vi "AddCalanderToFrontPanel.vi"() -> ()   [LabVIEW 2019]
panel:
  out "To Date  2":string
  out "To Date":string
  in  "To Date Time":timestamp
  in  "From Date Time":timestamp
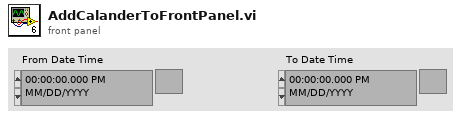
[diagram p1: front panel]
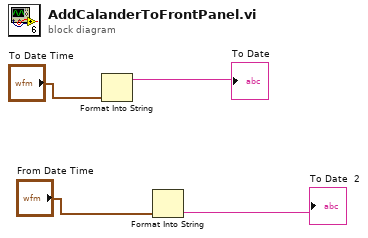
[diagram p0: block diagram]
diagram:
  n1 = Format Into String("To Date Time") -> (resulting string=→"To Date":string)  [unwired: 3 in, 1 out]
  n2 = Format Into String("From Date Time") -> (resulting string=→"To Date  2":string)  [unwired: 3 in, 1 out]
